vi "Hex to Normal String.vi"(11 "Hex String in":string) -> (3 "Normal String out":string)   [LabVIEW 2018, in "String Data Type.lvclass"]
uses:
  String Data Type.lvclass
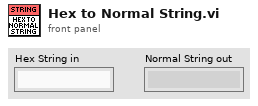
[diagram p1: front panel]
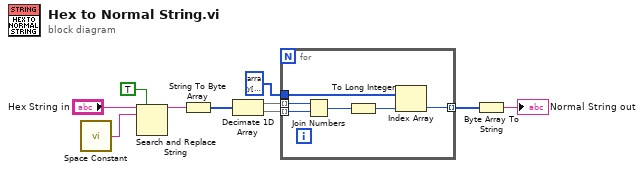
[diagram p0: block diagram]
diagram:
  n1 = call <vilib>:"Space Constant.vi"() -> ("String"=w2:string)
  n2 = Search and Replace String(replace all?=TRUE ("replace all? (F)"), input string="Hex String in", search string=w2) -> (result string=w8:string)  [unwired: 5 in, 3 out]
  n3 = String To Byte Array(string=w8) -> (unsigned byte array=w6:u8[])
  n4 = Decimate 1D Array(w6) -> (w5:u8[], w4:u8[])
  n5 = for {
    tunnel: [w16] -> w7 mode=indexing
    tunnel: w5 -> [w15] mode=indexing
    tunnel: w4 -> [w14] mode=indexing
    tunnel: u8[] array[65536 elements] ("Array") -> [w11]
    n6 = Join Numbers(hi=w15, lo=w14) -> ((hi.lo)=w13:u16)
    n7 = To Long Integer(number=w13) -> (32bit integer=w12:i32)
    n8 = Index Array(array=w11, index=w12) -> (element=w16:u8)
  }
  n9 = Byte Array To String(unsigned byte array=w7) -> (string=→"Normal String out":string)
